vi "Write Dev Motors with Brake Config.vi"(8 "error in (no error)":errorcluster, 10 "Dev Motors with Brake Config":T2={"Brake Set Channel"=enum."Invalid", "Pneumatics CAN ID"=0, "Brake Release Channel"=enum."Invalid"}, 11 "Dev Motors with Brake in":refnum<class "Dev Motors with Brake.lvclass">) -> (0 "error out":errorcluster, 3 "Dev Motors with Brake out":refnum<class "Dev Motors with Brake.lvclass">)   [LabVIEW 2014, in "Dev Motors with Brake.lvlib" / "Dev Motors with Brake.lvclass"]
uses:
  Dev Motors with Brake.lvclass
  <vilib>/Rock Robotics/WPI/Solenoid/WPI_SolenoidChannel.ctl
  Dev Motors with Brake.lvclass/Dev Motors with Brake.ctl
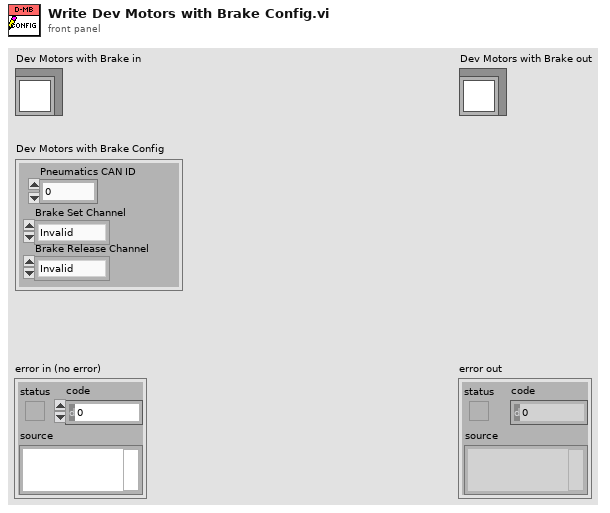
[diagram p1: front panel]
types:
  T1 = typedef "WPI_SolenoidChannel.ctl" = enum8{"Solenoid 0", "Solenoid 1", "Solenoid 2", "Solenoid 3", "Solenoid 4", "Solenoid 5", "Solenoid 6", "Solenoid 7", "Invalid"}
  T2 = cluster{"Brake Set Channel":T1, "Pneumatics CAN ID":u8, "Brake Release Channel":T1}
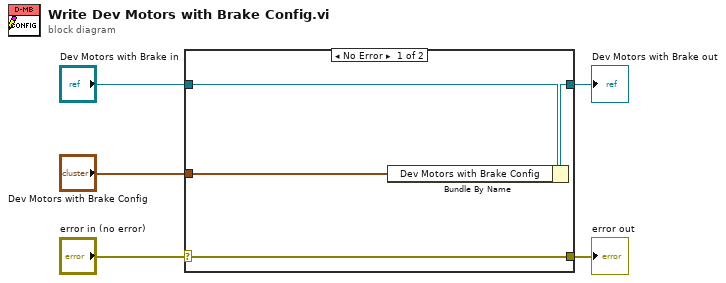
[diagram p0: block diagram]
diagram:
  n1 = case shown="No Error" "error in (no error)" {
    selector: "error in (no error)" -> [w9 w10]
    tunnel: [w9 w10] -> w4
    tunnel: [w7 w11] -> w2
    tunnel: "Dev Motors with Brake in" -> [w8 w11]
    tunnel: "Dev Motors with Brake Config" -> [w6 _]
    frame No Error {
      n2 = Bundle By Name(cluster=w8, "Dev Motors with Brake Config"=w6) -> (w7:refnum<class "Dev Motors with Brake.lvclass">)
    }
    frame Error {
    }
  }
  "error out" <- w4
  "Dev Motors with Brake out" <- w2
